vi "HexpSS(sous-VI).vi"(6 "Hexap_ON":bool, 9 "Playstation Button":bool, 10 "Stop_Hexap":refnum<vi>, 11 "Start_Hexap":refnum<vi>) -> ()   [LabVIEW 2019]
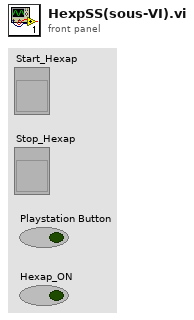
[diagram p1: front panel]
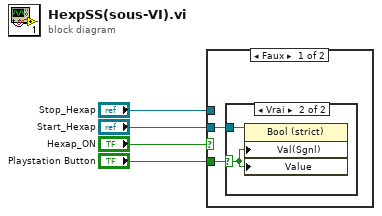
[diagram p0: block diagram]
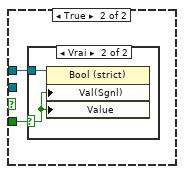
[diagram p3: hidden frame]
diagram:
  n1 = case shown="Faux" "Hexap_ON" {
    tunnel: "Playstation Button" -> [w5 w9]
    tunnel: "Start_Hexap" -> [w6 _]
    tunnel: "Stop_Hexap" -> [_ w10]
    frame False {
      n2 = case shown="Vrai" w5 {
        selector: w5 -> [_ w7]
        tunnel: w6 -> [_ w8]
        frame False {
        }
        frame True {
          n3 = property on="Nœud de propriété" class="Bool (strict)"(reference=w8, "Val(Sgnl)"=w7, "Value"=w7) -> ()  [unwired: 1 in, 2 out]
        }
      }
    }
    frame True {
      n4 = case shown="Vrai" w9 {
        selector: w9 -> [_ w11]
        tunnel: w10 -> [_ w12]
        frame False {
        }
        frame True {
          n5 = property on="Nœud de propriété" class="Bool (strict)"(reference=w12, "Val(Sgnl)"=w11, "Value"=w11) -> ()  [unwired: 1 in, 2 out]
        }
      }
    }
  }
